vi "SetHSV.vi"(0 "ColorHLS in":refnum<class "ColorHSV.lvclass">, 5 "H":dbl, 7 "S":dbl, 9 "V":dbl, 11 "error in (no error)":errorcluster) -> (4 "ColorHLS out":refnum<class "ColorHSV.lvclass">, 15 "error out":errorcluster)   [LabVIEW 2021, in "Picture2D.lvlib" / "ColorHSV.lvclass"]
uses:
  ColorHSV.lvclass
  ColorHSV.lvclass/ColorHSV.ctl
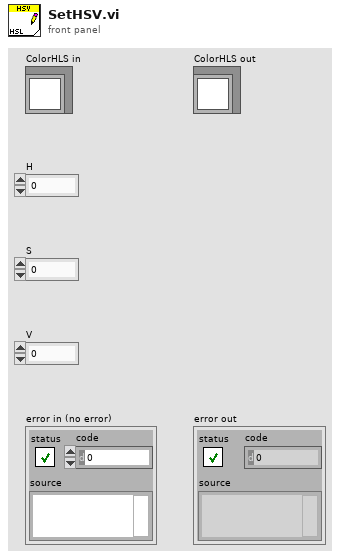
[diagram p1: front panel]
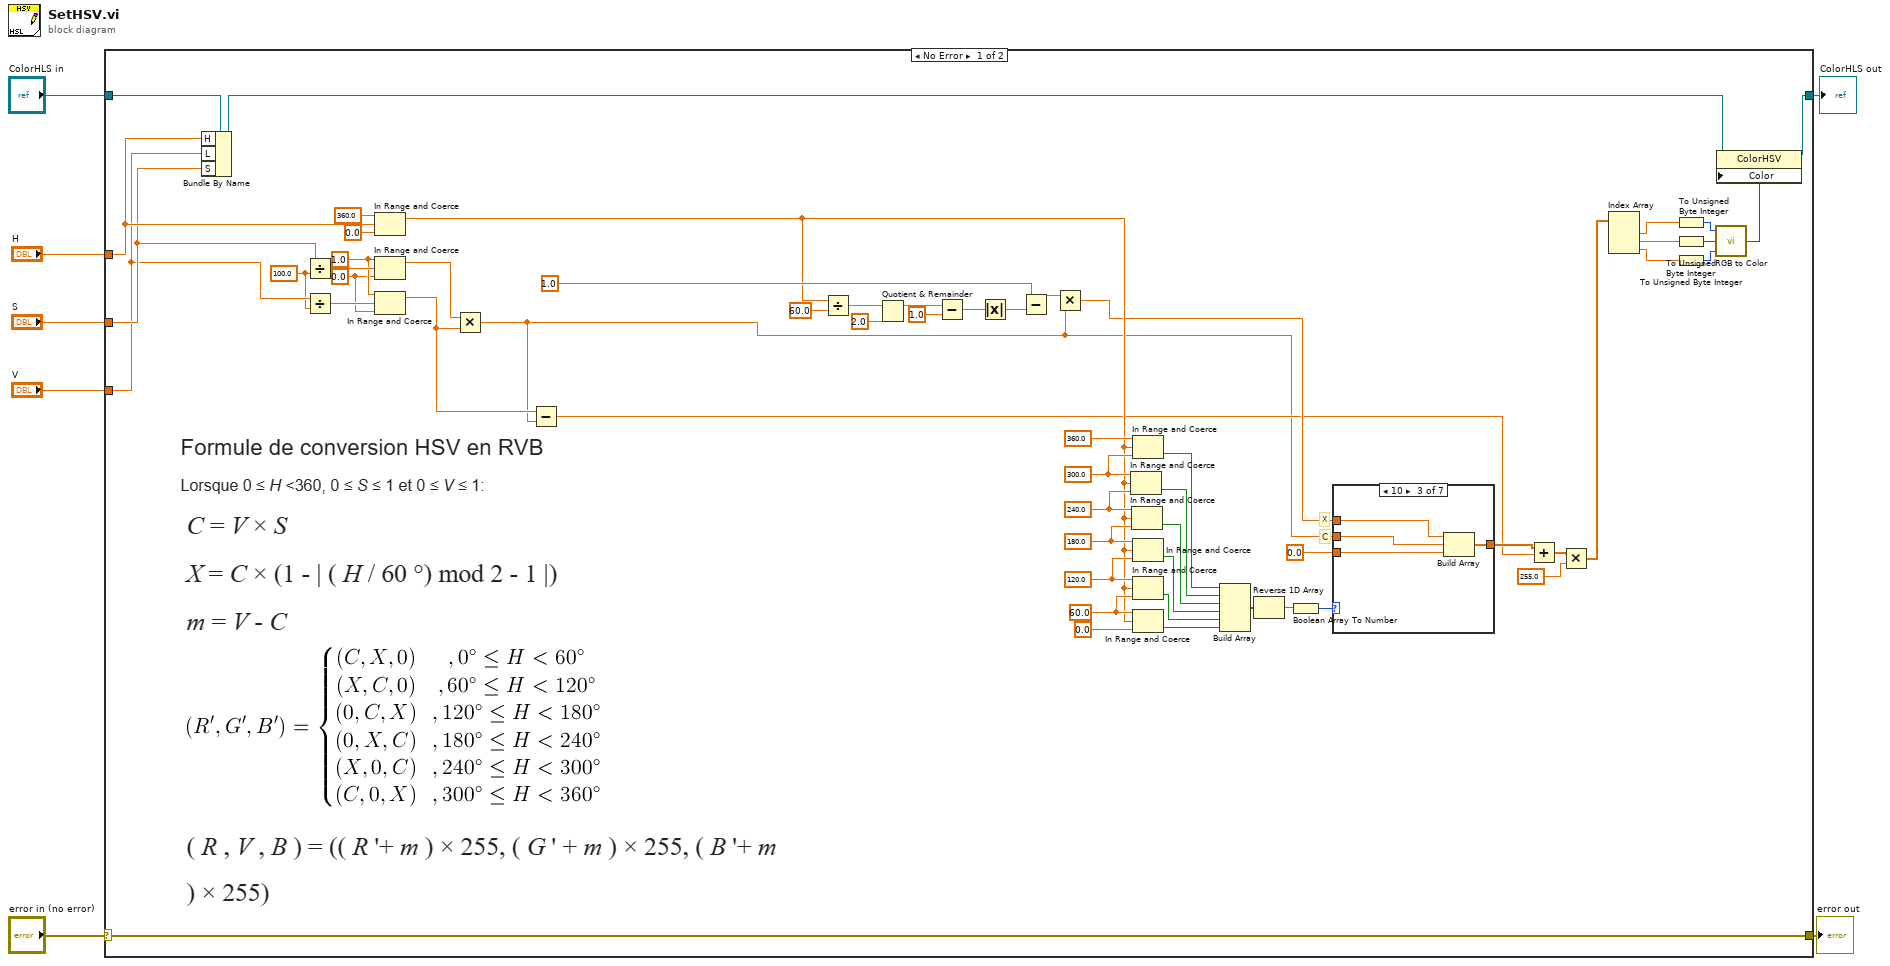
[diagram p0: block diagram]
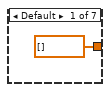
[diagram p2: hidden frame]
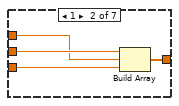
[diagram p3: hidden frame]
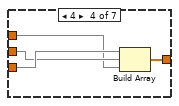
[diagram p4: hidden frame]
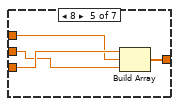
[diagram p5: hidden frame]
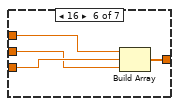
[diagram p6: hidden frame]
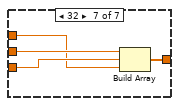
[diagram p7: hidden frame]
diagram:
  n1 = case shown="No Error" "error in (no error)" {
    selector: "error in (no error)" -> [w64 w90]
    tunnel: [w64 w90] -> w6
    tunnel: [w52 w91] -> w4
    tunnel: "ColorHLS in" -> [w63 w91]
    tunnel: "H" -> [w55 _]
    tunnel: "V" -> [w53 _]
    tunnel: "S" -> [w54 _]
    frame No Error {
      w26 = 300.0 ("upper limit")
      w27 = 240.0 ("upper limit")
      w28 = 180.0 ("upper limit")
      w29 = 120.0 ("upper limit")
      w31 = 60.0 ("upper limit")
      w44 = 0.0 ("lower limit")
      w45 = 1.0 ("upper limit")
      w50 = 100.0
      # "C"
      # "X"
      n2 = Bundle By Name(cluster=w63, "H"=w55, "L"=w53, "S"=w54) -> (w62:refnum<class "ColorHSV.lvclass">)
      n3 = Divide(x=w54, y=w50) -> (x/y=w47:dbl)
      n4 = Divide(x=w53, y=w50) -> (x/y=w46:dbl)
      n5 = In Range and Coerce(upper limit=360.0, x=w55, lower limit=0.0) -> (coerced(x)=w25:dbl)  [unwired: 1 out]
      n6 = In Range and Coerce(upper limit=w45, x=w47, lower limit=w44) -> (coerced(x)=w43:dbl)  [unwired: 1 out]
      n7 = In Range and Coerce(upper limit=w45, x=w46, lower limit=w44) -> (coerced(x)=w9:dbl)  [unwired: 1 out]
      n8 = Multiply(x=w43, y=w9) -> (x*y=w8:dbl)
      n9 = Subtract(x=w9, y=w8) -> (x-y=w13:dbl)
      n10 = Divide(x=w25, y=60.0) -> (x/y=w41:dbl)
      n11 = Quotient & Remainder(x=w41, y=2.0) -> (x-y*floor(x/y)=w39:dbl)  [unwired: 1 out]
      n12 = Subtract(x=w39, y=1.0) -> (x-y=w37:dbl)
      n13 = Absolute Value(x=w37) -> (abs(x)=w36:dbl)
      n14 = Subtract(x=1.0, y=w36) -> (x-y=w34:dbl)
      n15 = Multiply(x=w34, y=w8) -> (x*y=w16:dbl)
      n16 = In Range and Coerce(upper limit=w26, x=w25, lower limit=w27) -> (In Range?=w21:bool)  [unwired: 1 out]
      n17 = In Range and Coerce(upper limit=w27, x=w25, lower limit=w28) -> (In Range?=w22:bool)  [unwired: 1 out]
      n18 = In Range and Coerce(upper limit=360.0, x=w25, lower limit=w26) -> (In Range?=w20:bool)  [unwired: 1 out]
      n19 = In Range and Coerce(upper limit=w28, x=w25, lower limit=w29) -> (In Range?=w23:bool)  [unwired: 1 out]
      n20 = In Range and Coerce(upper limit=w29, x=w25, lower limit=w31) -> (In Range?=w24:bool)  [unwired: 1 out]
      n21 = In Range and Coerce(upper limit=w31, x=w25, lower limit=0.0) -> (In Range?=w33:bool)  [unwired: 1 out]
      n22 = Build Array(w20, w21, w22, w23, w24, w33) -> (w19:bool[])
      n23 = Reverse 1D Array(array=w19) -> (reversed array=w18:bool[])
      n24 = Boolean Array To Number(Boolean array=w18) -> (number=w17:u32)
      n25 = case shown="10" w17 {
        tunnel: w8 -> [_ w69 w73 w75 w78 w82 w87]
        tunnel: w16 -> [_ w68 w70 w74 w79 w84 w86]
        tunnel: 0.0 -> [_ w67 w72 w76 w80 w83 w88]
        tunnel: [dbl[] [] w66 w71 w77 w81 w85 w89] -> w14
        frame Default {
        }
        frame 1 {
          n26 = Build Array(w69, w68, w67) -> (w66:dbl[])
        }
        frame 2 {
          n27 = Build Array(w70, w73, w72) -> (w71:dbl[])
        }
        frame 4 {
          n28 = Build Array(w76, w75, w74) -> (w77:dbl[])
        }
        frame 8 {
          n29 = Build Array(w80, w79, w78) -> (w81:dbl[])
        }
        frame 16 {
          n30 = Build Array(w84, w83, w82) -> (w85:dbl[])
        }
        frame 32 {
          n31 = Build Array(w87, w88, w86) -> (w89:dbl[])
        }
      }
      n32 = Add(x=w14, y=w13) -> (x+y=w12:dbl[])
      n33 = Multiply(x=w12, y=255.0) -> (x*y=w10:dbl[])
      n34 = Index Array(array=w10) -> (element #1=w58:dbl, element #2=w57:dbl, element #3=w56:dbl)  [unwired: 3 in]
      n35 = To Unsigned Byte Integer(number=w58) -> (unsigned 8bit integer=w59:u8)
      n36 = To Unsigned Byte Integer(number=w57) -> (unsigned 8bit integer=w60:u8)
      n37 = To Unsigned Byte Integer(number=w56) -> (unsigned 8bit integer=w61:u8)
      n38 = call <vilib>:"RGB to Color.vi"("B"=w61, "G"=w60, "R"=w59) -> ("Color"=w51:u32)
      n39 = property class="ColorHSV"(reference=w62, "Color"=w51) -> (reference out=w52:refnum<class "ColorHSV.lvclass">)  [unwired: 1 in, 1 out]
    }
    frame Error {
    }
  }
  "error out" <- w6
  "ColorHLS out" <- w4
